vi "GetValueNumeric.vi"(7 "LabVIEW Web Service Request":refnum<class "Web Request.lvclass">, 11 "ControlName":string="Start") -> (1 "Error":i32, 2 "ErrorString":string, 3 "dataOut":dbl)   [LabVIEW 2024]
uses:
  <vilib>/wsapi/Web Request.lvclass
  g_VIServerPort.vi
panel:
  out "value":string
  out "errorOut":errorcluster
  # "Use the Web Service Request input terminal to call the VIs on the Web Services palette. Do not remove it from the connector pane unless you don't need access to the palette."
  # "Each additional control wired to the connector pane will be available as an input in the URL. To include an indicator in terminal-mode output (the default setting), it must also be wired to the connector pane."
  # "http://127.0.0.1:8080/WebService/GetValueNumeric?ControlName={value}"
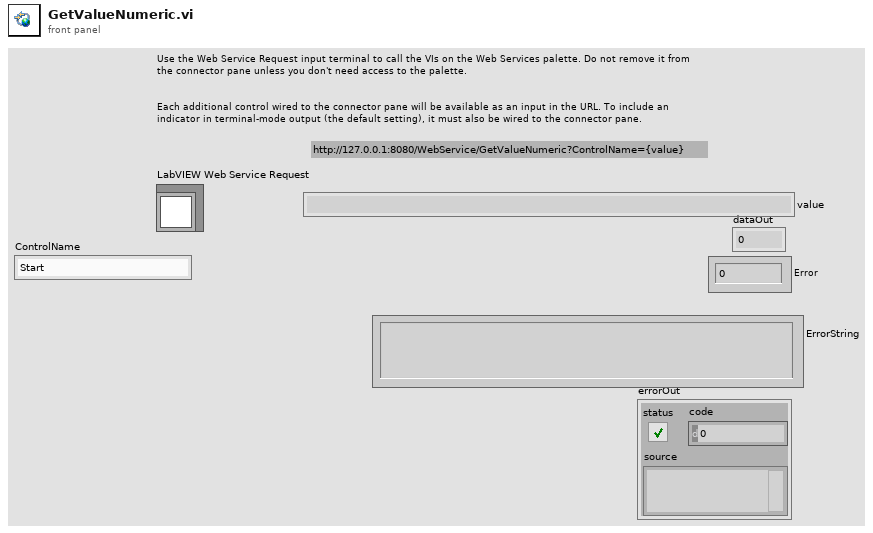
[diagram p1: front panel]
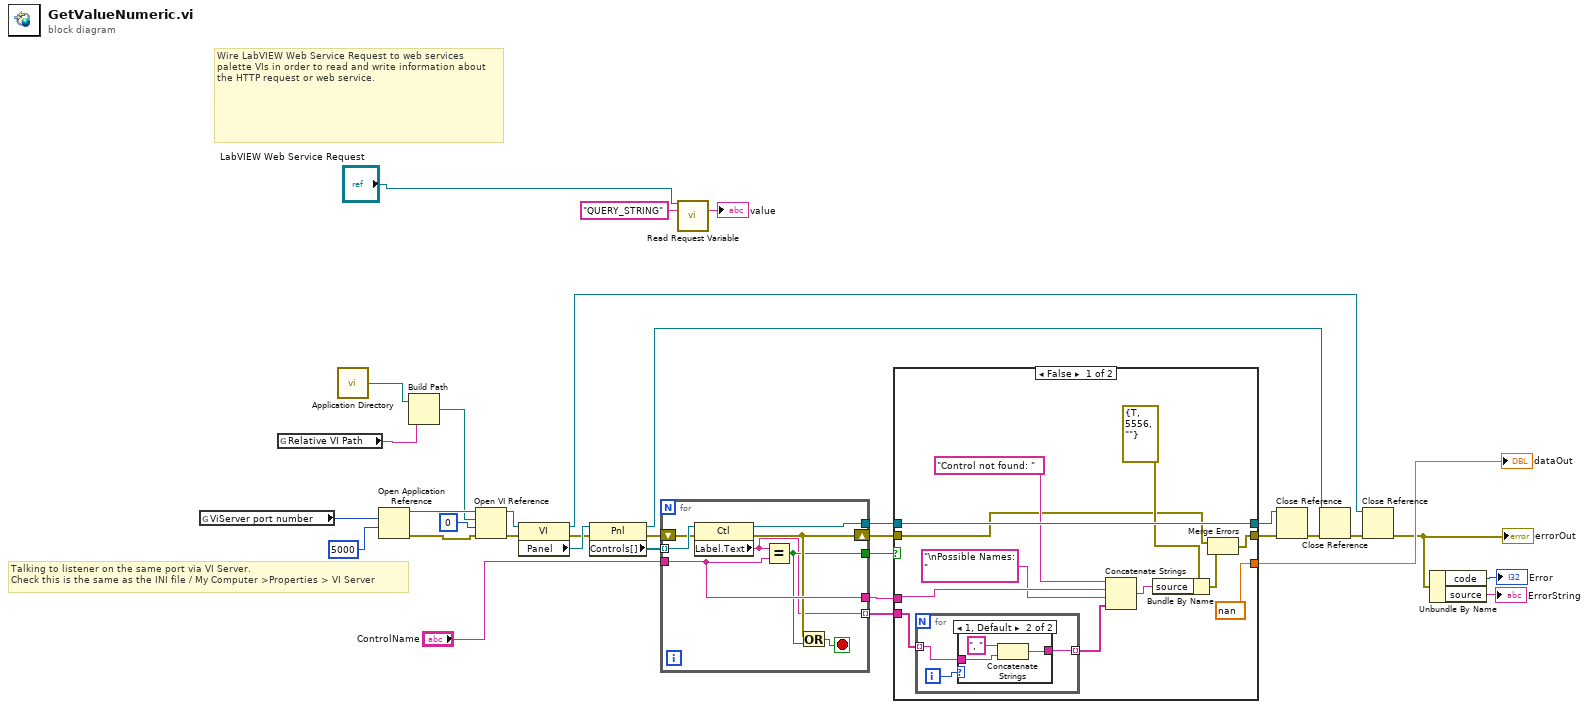
[diagram p0: block diagram]
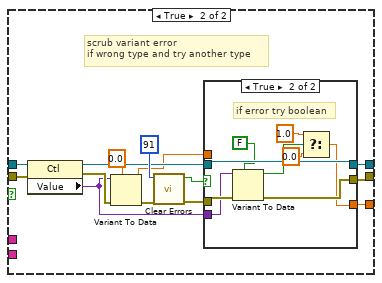
[diagram p3: hidden frame]
diagram:
  # "Talking to listener on the same port via VI Server.\nCheck this is the same as the INI file / My Computer >Properties > VI Server"
  # "Wire LabVIEW Web Service Request to web services palette VIs in order to read and write information about the HTTP request or web service."
  n1 = global read "g_VIServerPort.vi" "ViServer port number"() -> (w2:u16)
  n2 = global read "g_VIServerPort.vi" "Relative VI Path"() -> (w1:string)
  n3 = call <vilib>:"Application Directory.vi"() -> ("Application Directory"=w7:path)
  n4 = Open Application Reference(9:5000 ("timeout ms (60000)"), 10:w2) -> (0:w13:errorcluster, 3:w14:refnum<vi>)  [unwired: 2 in]
  n5 = Build Path(base path=w7, name or relative path=w1) -> (appended path=w6:path)
  n6 = Open VI Reference(application reference (local)=w14, vi path=w6, options=0, error in (no error)=w13) -> (vi reference=w17:refnum<vi>, error out=w29:errorcluster)  [unwired: 2 in]
  n7 = property class="VI"(reference=w17, error in=w29) -> (reference out=w24:refnum<vi>, error out=w28:errorcluster, "Panel"=w32:refnum<vi>)
  n8 = property class="Pnl"(reference=w32, error in=w28) -> (reference out=w18:refnum<vi>, error out=w27:errorcluster, "Controls[]"=w31:refnum<vi>[])
  n9 = for {
    tunnel: w31 -> [w41] mode=indexing
    tunnel: "ControlName" -> [w38]
    tunnel: [w35] -> w26
    tunnel: [w39] -> w19
    tunnel: [w38] -> w15
    shift-right: [w36] -> w20
    shift-left: w27 -> [w40]
    tunnel: [w34] -> w9 mode=indexing
    stop <- w37 stop-if-true
    n10 = property class="Ctl"(reference=w41, error in=w40) -> (reference out=w39:refnum<vi>, error out=w36:errorcluster, "Label.Text"=w34:string)
    n11 = Equal?(x=w34, y=w38) -> (x = y?=w35:bool)
    n12 = Or(x=w36, y=w35) -> (x .or. y?=w37:bool)
  }
  n13 = call <vilib>:"Read Request Variable.vi"("LabVIEW Web Service Request"="LabVIEW Web Service Request", "variable name"="QUERY_STRING") -> ("value"=→"value":string)  [unwired: 11 in, 2 out]
  n14 = case shown="False" w26 {
    tunnel: w19 -> [w53 w74]
    tunnel: [w53 w69] -> w25
    tunnel: [w47 w68] -> w21
    tunnel: w20 -> [w48 w73]
    tunnel: [nan ("Ctrl Val to set (Num)") w62] -> w16
    tunnel: w15 -> [w45 _]
    tunnel: w9 -> [w43 _]
    frame False {
      n15 = for {
        tunnel: w43 -> [w54] mode=indexing
        tunnel: [w56] -> w42 mode=indexing
        i -> [w55]
        n16 = case shown="1, Default" w55 {
          tunnel: [w57 w60] -> w56
          tunnel: w54 -> [w57 w58]
          frame 0 {
          }
          frame 1, Default {
            n17 = Concatenate Strings(", " ("string"), w58) -> (w60:string)
          }
        }
      }
      n18 = Concatenate Strings("Control not found: " ("string"), w45, "\nPossible Names: " ("string"), w42) -> (w51:string)
      n19 = Bundle By Name(cluster=errorcluster {"status"=TRUE, "code"=5556, "source"=""} ("error constant"), "source"=w51) -> (w49:errorcluster)
      n20 = Merge Errors(w48, w49) -> (w47:errorcluster)
    }
    frame True {
      # "scrub variant error\nif wrong type and try another type"
      n21 = property class="Ctl"(reference=w74, error in=w73) -> (reference out=w70:refnum<vi>, error out=w64:errorcluster, "Value"=w63:variant)
      n22 = Variant To Data(error in=w64, type=0.0 ("Ctrl Val to set (Num)"), Variant=w63) -> (data=w61:dbl, error out=w65:errorcluster)
      n23 = call <vilib>:"Clear Errors.vi"("error in (no error)"=w65, "specific error code to clear (0: all)"=91) -> ("error out"=w67:errorcluster, "specific error cleared?"=w71:bool)  [unwired: 4 in]
      n24 = case shown="True" w71 {
        tunnel: w70 -> [w77 w86]
        tunnel: [w77 w86] -> w69
        tunnel: [w76 w83] -> w68
        tunnel: w67 -> [w76 w85]
        tunnel: w63 -> [_ w84]
        tunnel: [w75 w80] -> w62
        tunnel: w61 -> [w75 _]
        frame False {
        }
        frame True {
          # "if error try boolean"
          n25 = Variant To Data(error in=w85, type=FALSE, Variant=w84) -> (data=w81:bool, error out=w83:errorcluster)
          n26 = Select(t=1.0, s=w81, f=0.0) -> (s? t:f=w80:dbl)
        }
      }
    }
  }
  "dataOut" <- w16
  n27 = Close Reference(reference=w25, error in (no error)=w21) -> (error out=w23:errorcluster)
  n28 = Close Reference(reference=w18, error in (no error)=w23) -> (error out=w22:errorcluster)
  n29 = Close Reference(reference=w24, error in (no error)=w22) -> (error out=w12:errorcluster)
  "errorOut" <- w12
  n30 = Unbundle By Name(w12) -> ("code"=→"Error":i32, "source"=→"ErrorString":string)
